vi "Panel Resize.vi"(6 "Control Ref Queue":T1, 8 "error in (no error)":errorcluster, 11 "3D Plot.lvclass":refnum<class "3D Plot.lvclass">) -> (0 "error out":errorcluster, 3 "3D Plot.lvclass out":refnum<class "3D Plot.lvclass">)   [LabVIEW 2020, in "3D Plot.lvclass"]
uses:
  <vilib>/Math Plots/3D Math Plots/3D Plot/3D Plot/3D Plot.lvclass
  <vilib>/Math Plots/3D Math Plots/3D Plot/Action String/3DMathPlot Ctrl Act Queue.ctl
  <vilib>/Math Plots/3D Math Plots/3D Plot/Action String/3DMathPlot Ctrl Act Cluster.ctl
  <vilib>/Math Plots/3D Math Plots/3D Plot/Action String/3DMathPlot State Class.ctl
  <vilib>/Math Plots/3D Math Plots/3D Plot/3D Plot/3D Plot.lvclass/3D Plot.ctl
  <vilib>/Math Plots/Plot Private Lib/NI_Math Plot Private Lib.lvlib
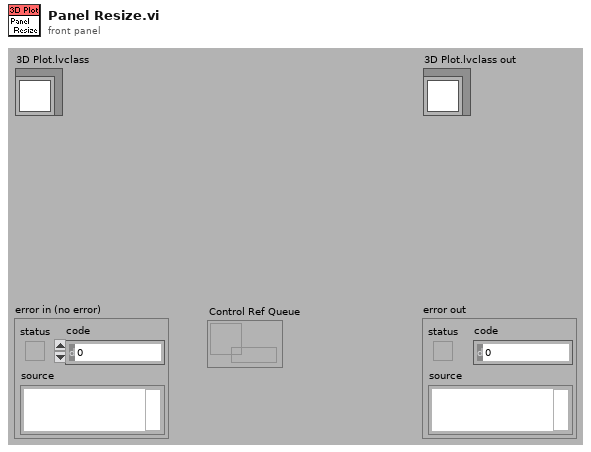
[diagram p1: front panel]
types:
  T1 = typedef "3DMathPlot Ctrl Act Queue.ctl" = refnum<queue>
  T2 = typedef "3DMathPlot Ctrl Act Cluster.ctl" = cluster{"3D Picture Control":refnum<vi>, "Render Window Refnum":refnum<vi>, "XY Graph":refnum<vi>, "Intensity Graph":refnum<vi>, "Color Legend Palette":refnum<vi>, "Projection Palette":refnum<vi>, "XControl  Ref":refnum<vi>, "Facade Ref":refnum<vi>, "Export Image Ref":refnum<vi>, "Clear Data Flag":bool, "Display State Change Class":T3}
  T3 = typedef "3DMathPlot State Class.ctl" = enum16{"Update All Objects (Undo)", "Update Light Object Only", "Update Axis Object Only", "Update Plot Object Only", "Update Cursor Object Only", "Update Axis Plot Cursor Objects", "No Update"}
  T4 = enum32{"Towards X-Y Plane", "Towards X-Z Plane", "Towards Y-Z Plane", "User Defined"}
  T5 = typedef "LVPositionTypeDef.ctl" = cluster{"Left":i32, "Top":i32}
  T6 = typedef "LVRectTypeDef.ctl" = cluster{"Left":i16, "Top":i16, "Right":i16, "Bottom":i16}
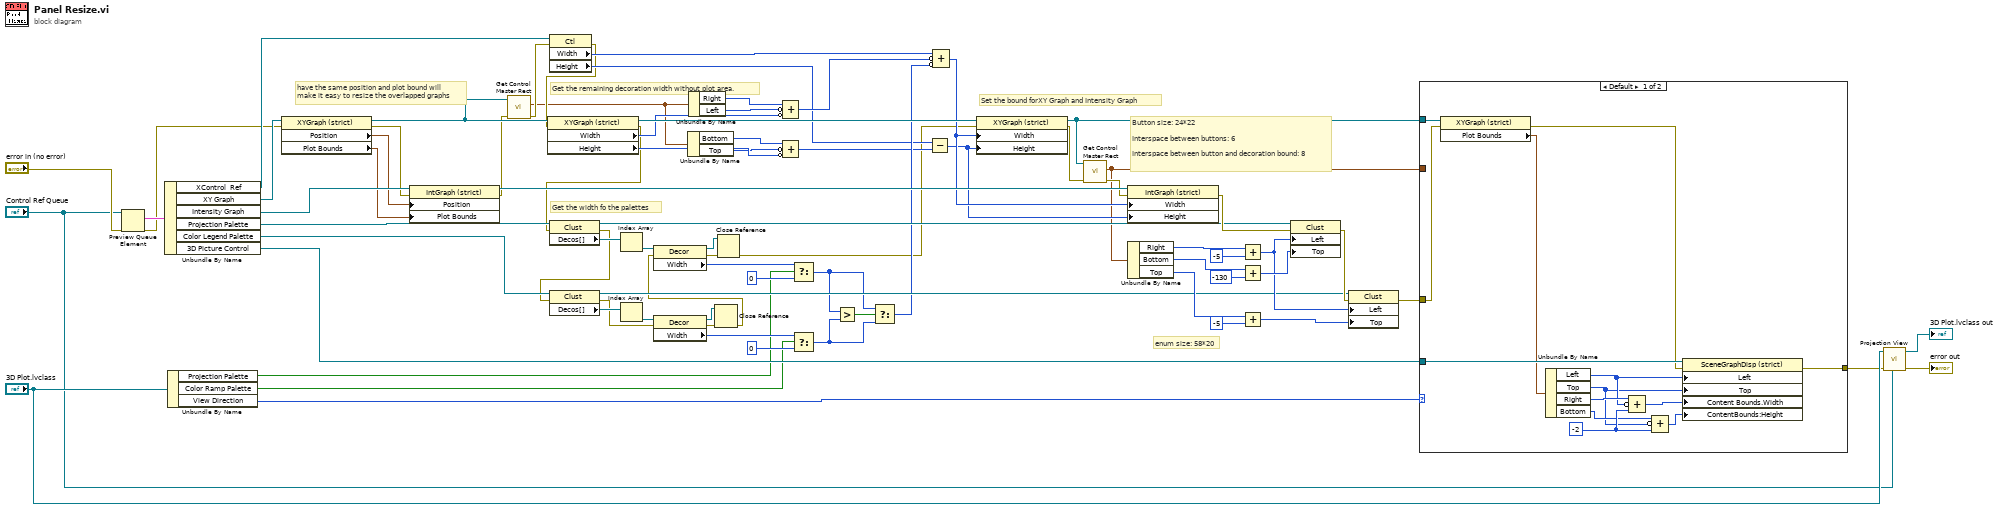
[diagram p0: block diagram]
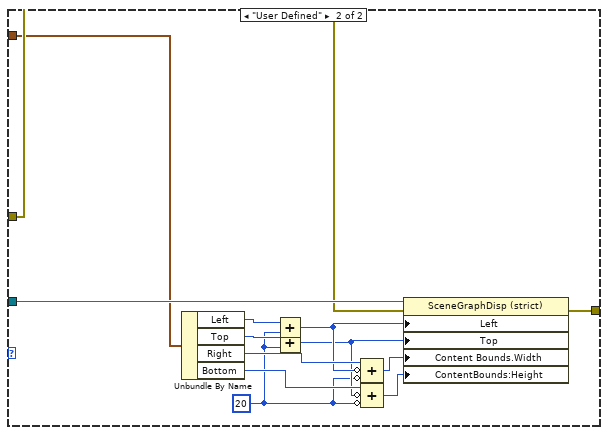
[diagram p2: hidden frame]
diagram:
  # "Set the bound forXY Graph and Intensity Graph"
  # "Get the remaining decoration width without plot area."
  # "Get the width fo the palettes"
  # "have the same position and plot bound will \nmake it easy to resize the overlapped graphs"
  # "enum size: 58*20"
  # "Button size: 24*22\n\nInterspace between buttons: 6\n\nInterspace between button and decoration bound: 8"
  n1 = Preview Queue Element(queue="Control Ref Queue", error in (no error)="error in (no error)") -> (element=w39:T2, error out=w30:errorcluster)  [unwired: 3 out]
  n2 = Unbundle By Name(w39) -> ("XControl  Ref"=w61:refnum<vi>, "XY Graph"=w34:refnum<vi>, "Intensity Graph"=w36:refnum<vi>, "Projection Palette"=w54:refnum<vi>, "Color Legend Palette"=w57:refnum<vi>, "3D Picture Control"=w60:refnum<vi>)
  n3 = Unbundle By Name("3D Plot.lvclass") -> ("Projection Palette"=w38:bool, "Color Ramp Palette"=w37:bool, "View Direction"=w59:T4)
  n4 = property on="Property Node" class="XYGraph (strict)"(reference=w34, error in=w30) -> (reference out=w16:refnum<vi>, error out=w31:errorcluster, "Position"=w33:T5, "Plot Bounds"=w32:T6)
  n5 = property on="Property Node" class="IntGraph (strict)"(reference=w36, error in=w31, "Position"=w33, "Plot Bounds"=w32) -> (reference out=w35:refnum<vi>, error out=w15:errorcluster)
  n6 = call <vilib>:"Get Control Master Rect.vi"("error in (no error)"=w15, "reference"=w16) -> ("error out"=w14:errorcluster, "Master Bounds Rect"=w11:T6)  [unwired: 8 out]
  n7 = property on="Property Node" class="Ctl"(reference=w61, error in=w14) -> (error out=w13:errorcluster, "Width"=w62:u32, "Height"=w21:u32)  [unwired: 1 out]
  n8 = property on="Property Node" class="XYGraph (strict)"(reference=w16, error in=w13) -> (reference out=w29:refnum<vi>, error out=w12:errorcluster, "Width"=w26:u32, "Height"=w22:u32)
  n9 = property on="Property Node" class="Clust"(reference=w54, error in=w12) -> (reference out=w53:refnum<vi>, error out=w42:errorcluster, "Decos[]"=w52:refnum<vi>[])
  n10 = property on="Property Node" class="Clust"(reference=w57, error in=w42) -> (reference out=w56:refnum<vi>, error out=w40:errorcluster, "Decos[]"=w46:refnum<vi>[])
  n11 = Index Array(array=w52) -> (element=w51:refnum<vi>)  [unwired: 1 in]
  n12 = Index Array(array=w46) -> (element=w41:refnum<vi>)  [unwired: 1 in]
  n13 = property on="Property Node" class="Decor"(reference=w41, error in=w40) -> (reference out=w3:refnum<vi>, error out=w2:errorcluster, "Width"=w47:u32)
  n14 = Unbundle By Name(w11) -> ("Bottom"=w19:i16, "Top"=w18:i16)
  n15 = Unbundle By Name(w11) -> ("Right"=w28:i16, "Left"=w27:i16)
  n16 = Close Reference(reference=w3, error in (no error)=w2) -> (error out=w1:errorcluster)
  n17 = property on="Property Node" class="Decor"(reference=w51, error in=w1) -> (reference out=w6:refnum<vi>, error out=w5:errorcluster, "Width"=w50:u32)
  n18 = Close Reference(reference=w6, error in (no error)=w5) -> (error out=w4:errorcluster)
  n19 = Compound Arithmetic op=ADD(w28, invert w27, invert w26) -> (w25:u32)
  n20 = Compound Arithmetic op=ADD(w19, invert w18, invert w22) -> (w20:u32)
  n21 = Select(t=w50, s=w38, f=u32 0) -> (s? t:f=w44:u32)
  n22 = Select(t=w47, s=w37, f=u32 0) -> (s? t:f=w43:u32)
  n23 = Greater?(x=w44, y=w43) -> (0:w45:bool)
  n24 = Select(t=w44, s=w45, f=w43) -> (s? t:f=w24:u32)
  n25 = Subtract(x=w21, y=w20) -> (x-y=w17:u32)
  n26 = Compound Arithmetic op=ADD(w62, invert w25, invert w24) -> (w23:u32)
  n27 = property on="Property Node" class="XYGraph (strict)"(reference=w29, error in=w4, "Width"=w23, "Height"=w17) -> (reference out=w10:refnum<vi>, error out=w9:errorcluster)
  n28 = call <vilib>:"Get Control Master Rect.vi"("error in (no error)"=w9, "reference"=w10) -> ("error out"=w8:errorcluster, "Master Bounds Rect"=w7:T6)  [unwired: 8 out]
  n29 = property on="Property Node" class="IntGraph (strict)"(reference=w35, error in=w8, "Width"=w23, "Height"=w17) -> (error out=w55:errorcluster)  [unwired: 1 out]
  n30 = Unbundle By Name(w7) -> ("Right"=w66:i16, "Bottom"=w72:i16, "Top"=w65:i16)
  n31 = Add(x=w66, y=i16 -5) -> (x+y=w64:i16)
  n32 = Add(x=w72, y=i16 -130) -> (x+y=w67:i16)
  n33 = Add(x=w65, y=i16 -5) -> (x+y=w69:i16)
  n34 = property on="Property Node" class="Clust"(reference=w53, error in=w55, "Left"=w64, "Top"=w67) -> (error out=w63:errorcluster)  [unwired: 1 out]
  n35 = property on="Property Node" class="Clust"(reference=w56, error in=w63, "Left"=w64, "Top"=w69) -> (error out=w58:errorcluster)  [unwired: 1 out]
  n36 = case shown="Default" w59 {
    tunnel: w60 -> [w91 w100]
    tunnel: w10 -> [w90 _]
    tunnel: w58 -> [w88 w93]
    tunnel: [w87 w95] -> w75
    tunnel: w7 -> [_ w92]
    frame Default {
      w86 = i16 -2
      n37 = property on="Property Node" class="XYGraph (strict)"(reference=w90, error in=w88) -> (error out=w89:errorcluster, "Plot Bounds"=w83:T6)  [unwired: 1 out]
      n38 = Unbundle By Name(w83) -> ("Left"=w82:i16, "Top"=w81:i16, "Right"=w84:i16, "Bottom"=w85:i16)
      n39 = Compound Arithmetic op=ADD(w84, invert w82, w86) -> (w80:i16)
      n40 = Compound Arithmetic op=ADD(w85, invert w81, w86) -> (w79:i16)
      n41 = property class="SceneGraphDisp (strict)"(reference=w91, error in=w89, "Left"=w82, "Top"=w81, "Content Bounds.Width"=w80, "ContentBounds:Height"=w79) -> (error out=w87:errorcluster)  [unwired: 1 out]
    }
    frame "User Defined" {
      w94 = i16 20 ("y")
      n42 = Unbundle By Name(w92) -> ("Left"=w102:i16, "Top"=w103:i16, "Right"=w101:i16, "Bottom"=w104:i16)
      n43 = Add(x=w102, y=w94) -> (x+y=w99:i16)
      n44 = Add(x=w103, y=w94) -> (x+y=w98:i16)
      n45 = Compound Arithmetic op=ADD(w101, invert w99, invert w94) -> (w97:i16)
      n46 = Compound Arithmetic op=ADD(w104, invert w98, invert w94) -> (w96:i16)
      n47 = property class="SceneGraphDisp (strict)"(reference=w100, error in=w93, "Left"=w99, "Top"=w98, "Content Bounds.Width"=w97, "ContentBounds:Height"=w96) -> (error out=w95:errorcluster)  [unwired: 1 out]
    }
  }
  n48 = call <vilib>:"Projection View.vi"("Control Ref Queue"="Control Ref Queue", "error in (no error)"=w75, "3D Plot.lvclass in"="3D Plot.lvclass") -> ("error out"=→"error out":errorcluster, "3D Plot.lvclass out"=→"3D Plot.lvclass out":refnum<class "3D Plot.lvclass">)  [unwired: 1 in, 6 out]
